vi "GreeterService GetFeature.vi"(3 "error in (no error)":errorcluster, 4 "gRPCid in":T1, 5 "DNL_LabVIEW Object in":refnum<class "GreeterServiceImpl.lvclass">) -> (0 "error out":errorcluster, 1 "gRPCid out":T1, 2 "DNL_LabVIEW Object out":refnum<class "GreeterServiceImpl.lvclass">)   [LabVIEW 2019, in "UserCode_server.lvlib" / "GreeterServiceImpl.lvclass"]
uses:
  GreeterServiceImpl.lvclass
  <vilib>/gRPC/LabVIEW gRPC Library/Shared/grpcId.ctl
  Generated_server/RPC Messages/Greeter_res.ctl
  Generated_server/RPC Messages/Greeter_res_res_oneof/Greeter_res_res_oneof.lvclass
  Generated_server/RPC Messages/Greeter_MessageA.ctl
  Generated_server/RPC Messages/Greeter_req_req_oneof/Greeter_req_req_oneof.lvclass/Greeter_req_req_oneof.ctl
  Generated_server/RPC Messages/Greeter_res_res_oneof/Greeter_res_res_oneof.lvclass/Greeter_res_res_oneof.ctl
  Generated_server/RPC Service/GreeterService/GreeterService.lvclass
  Generated_server/RPC Messages/Greeter_req_req_oneof/Greeter_req_req_oneof.lvclass
  Generated_server/Generated_server.lvlib
  <vilib>/gRPC/LabVIEW gRPC Library/grpc-lvsupport-release.lvlib
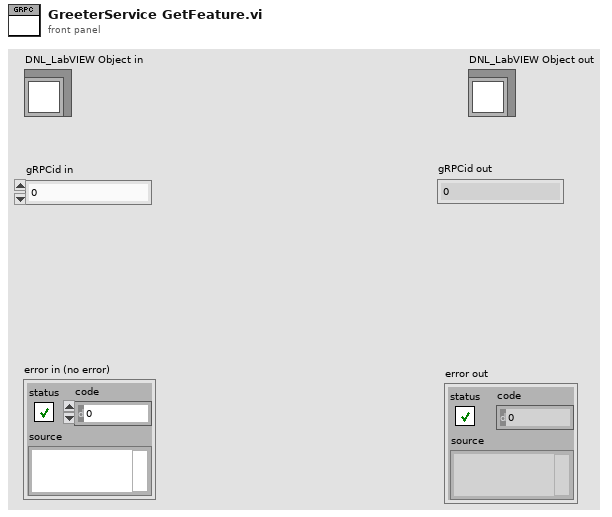
[diagram p1: front panel]
types:
  T1 = typedef "grpc-lvsupport-release.lvlib/grpcId.ctl" = u64
  T2 = typedef "Generated_server.lvlib/Greeter_res.ctl" = cluster{"res_latitude":i32, "Greeter_res_res_oneof":refnum<class "Greeter_res_res_oneof.lvclass">, "message_a":T3}
  T3 = typedef "Generated_server.lvlib/Greeter_MessageA.ctl" = cluster{"data_a1":string}
  T4 = typedef "Generated_server.lvlib/Greeter_req.ctl" = cluster{"req_latitude":i32, "message_a":T3, "Greeter_req_req_oneof":refnum<class "Greeter_req_req_oneof.lvclass">}
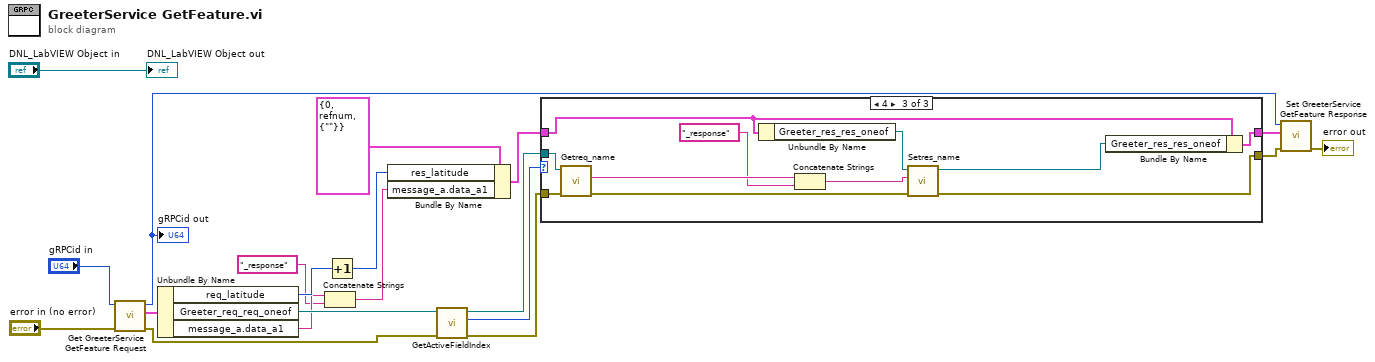
[diagram p0: block diagram]
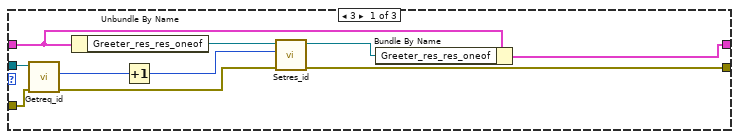
[diagram p2: hidden frame]
diagram:
  n1 = call "Get GreeterService GetFeature Request.vi"("error in (no error)"="error in (no error)", "gRPCid"="gRPCid in") -> ("error out"=w9:errorcluster, "Message Data"=w20:T4, "gRPCid out"=w1:T1)  [unwired: 7 in]
  "gRPCid out" <- w1
  n2 = Unbundle By Name(w20) -> ("req_latitude"=w15:i32, "Greeter_req_req_oneof"=w19:refnum<class "Greeter_req_req_oneof.lvclass">, "message_a.data_a1"=w12:string)
  n3 = Concatenate Strings(w12, "_response" ("string")) -> (w11:string)
  n4 = Increment(x=w15) -> (x+1=w14:i32)
  n5 = Bundle By Name(cluster=T2 {"res_latitude"=0, "Greeter_res_res_oneof"=refnum, "message_a"={"data_a1"=""}} ("Greeter_res"), "res_latitude"=w14, "message_a.data_a1"=w11) -> (w13:T2)
  n6 = call "GetActiveFieldIndex.vi"("error in (no error)"=w9, "OneOfTemplate in"=w19) -> ("error out"=w7:errorcluster, "Active Field Index"=w18:i32, "OneOfTemplate out"=w17:refnum<class "Greeter_req_req_oneof.lvclass">)  [unwired: 7 in]
  n7 = case shown="4" w18 {
    tunnel: w13 -> [w30 w32 w39]
    tunnel: w17 -> [w27 _ w43]
    tunnel: [w29 w32 w36] -> w8
    tunnel: w7 -> [w28 w31 w35]
    tunnel: [w21 w31 w33] -> w6
    frame 3 {
      n8 = call "Getreq_id.vi"("error in (no error)"=w28, "OneOfTemplate in"=w27) -> ("error out"=w26:errorcluster, "Get_Val"=w25:i32)  [unwired: 7 in, 1 out]
      n9 = Unbundle By Name(w30) -> ("Greeter_res_res_oneof"=w23:refnum<class "Greeter_res_res_oneof.lvclass">)
      n10 = Increment(x=w25) -> (x+1=w24:i32)
      n11 = call "Setres_id.vi"("error in (no error)"=w26, "Set_Val"=w24, "OneOfTemplate in"=w23) -> ("error out"=w21:errorcluster, "OneOfTemplate out"=w22:refnum<class "Greeter_res_res_oneof.lvclass">)  [unwired: 7 in]
      n12 = Bundle By Name(cluster=w30, "Greeter_res_res_oneof"=w22) -> (w29:T2)
    }
    frame 0, Default {
    }
    frame 4 {
      n13 = call "Getreq_name.vi"("error in (no error)"=w35, "OneOfTemplate in"=w43) -> ("error out"=w34:errorcluster, "Get_Val"=w42:string)  [unwired: 7 in, 1 out]
      n14 = Unbundle By Name(w39) -> ("Greeter_res_res_oneof"=w38:refnum<class "Greeter_res_res_oneof.lvclass">)
      n15 = Concatenate Strings(w42, "_response" ("string")) -> (w40:string)
      n16 = call "Setres_name.vi"("error in (no error)"=w34, "Set_Val"=w40, "OneOfTemplate in"=w38) -> ("error out"=w33:errorcluster, "OneOfTemplate out"=w37:refnum<class "Greeter_res_res_oneof.lvclass">)  [unwired: 7 in]
      n17 = Bundle By Name(cluster=w39, "Greeter_res_res_oneof"=w37) -> (w36:T2)
    }
  }
  n18 = call "Set GreeterService GetFeature Response.vi"("error in (no error)"=w6, "Message Data"=w8, "gRPCid in"=w1) -> ("error out"=→"error out":errorcluster)  [unwired: 8 in]
  "DNL_LabVIEW Object out" <- "DNL_LabVIEW Object in"
